vi "Set Test Finder.vi"(8 "error in (no error)":errorcluster, 11 "Execution Profiler In":refnum<class "Execution Profiler.lvclass">) -> (0 "error out":errorcluster, 3 "Execution Profiler Out":refnum<class "Execution Profiler.lvclass">)   [LabVIEW 2020, in "Execution Profiler.lvlib" / "Execution Profiler.lvclass"]
uses:
  Execution Profiler.lvclass
  C:/git/astemes-lunit/source/User Interface/Process/Process.lvclass
  User Interface/Process/Process.lvclass/Process.ctl
  User Interface/Process/Process.lvclass
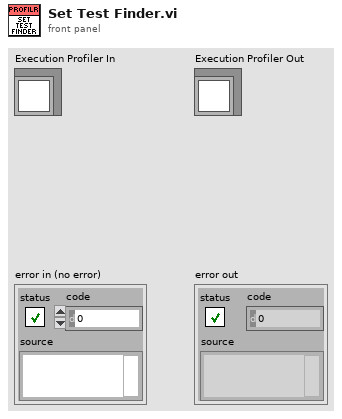
[diagram p1: front panel]
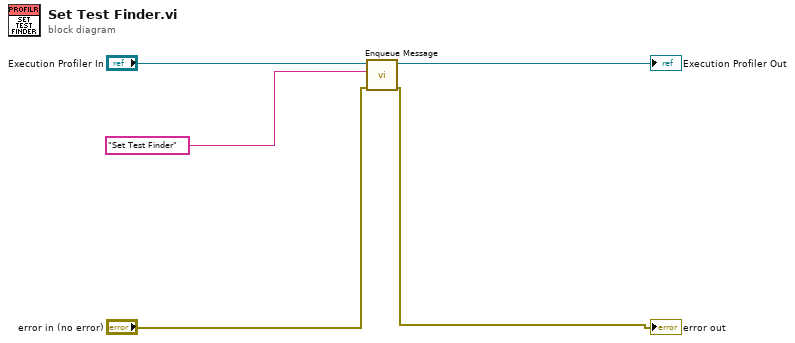
[diagram p0: block diagram]
diagram:
  n1 = call "Enqueue Message.vi"("error in (no error)"="error in (no error)", "Message"="Set Test Finder", "Process In"="Execution Profiler In") -> ("error out"=→"error out":errorcluster, "Process Out"=→"Execution Profiler Out":refnum<class "Execution Profiler.lvclass">)  [unwired: 7 in]
